vi "Iterate Owned Items.vi"(8 "Error In":errorcluster, 10 "Owned Items[]":refnum<vi>[](array[refnum]), 11 "Project Items In":T1[](array[typedef])) -> (0 "Error Out":errorcluster, 3 "Project Items Out":T1[](array[typedef]))   [LabVIEW 2014, in "i3-docs.lvlib"]
uses:
  i3-docs.lvlib
  Controls/project_item.ctl
  Controls/image_information.ctl
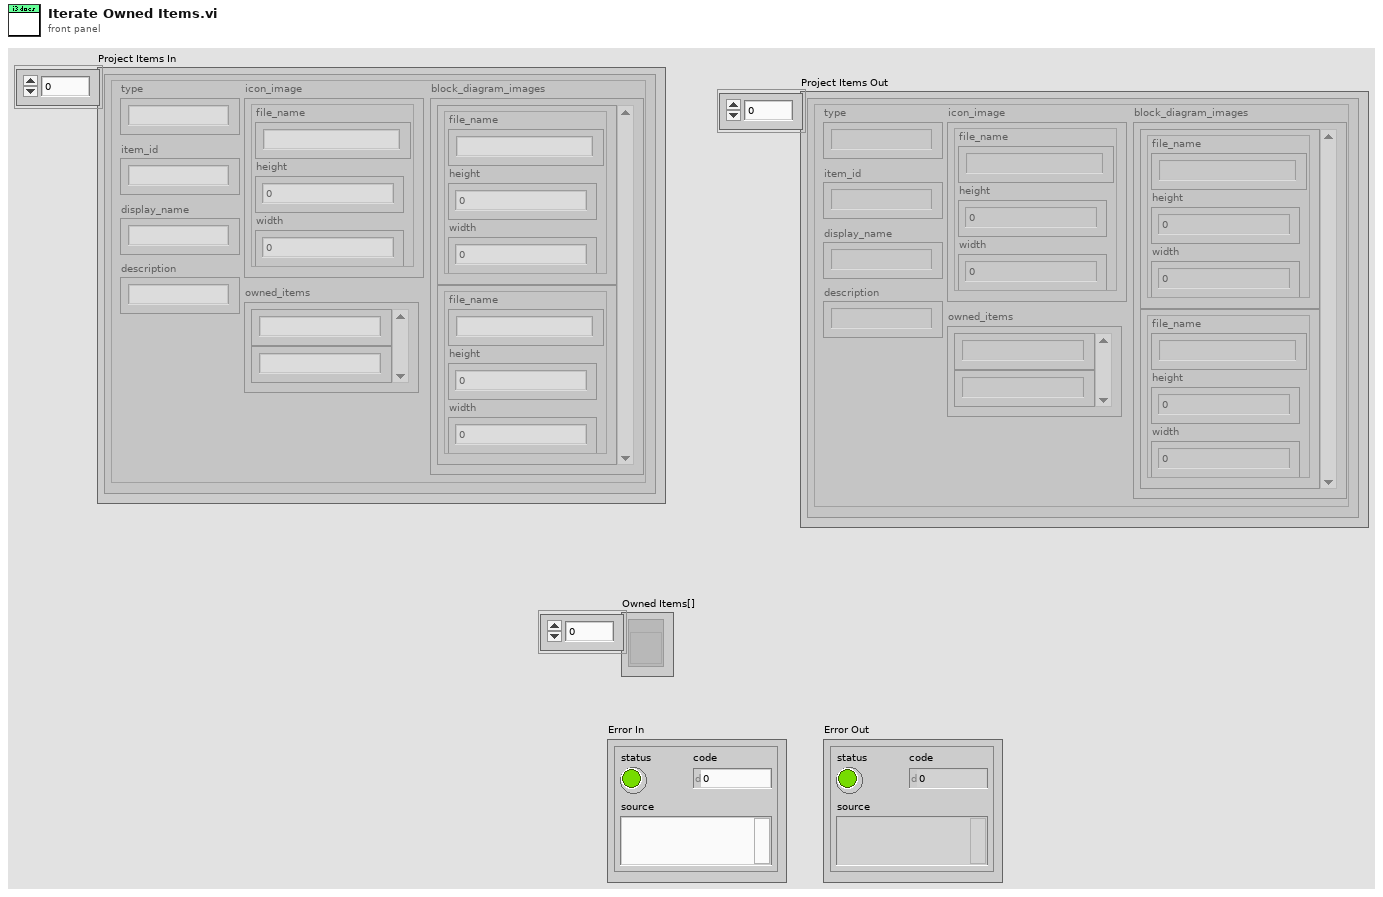
[diagram p1: front panel]
types:
  T1 = typedef "i3-docs.lvlib/project_item.ctl" = cluster{"type":string, "owned_items":string[], "item_id":string, "display_name":string, "description":string, "block_diagram_images":T2[], "icon_image":T2}
  T2 = typedef "i3-docs.lvlib/image_information.ctl" = cluster{"file_name":string, "height":i32, "width":i32}
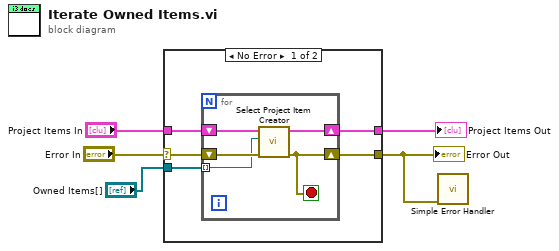
[diagram p0: block diagram]
diagram:
  n1 = case shown="No Error" "Error In" {
    selector: "Error In" -> [w10 w16]
    tunnel: "Project Items In" -> [w9 w17]
    tunnel: [w8 w16] -> w1
    tunnel: [w7 w17] -> w3
    tunnel: "Owned Items[]" -> [w6 _]
    frame No Error {
      n2 = for {
        tunnel: w6 -> [w11] mode=indexing
        shift-right: [w13] -> w8
        shift-left: w10 -> [w12]
        shift-right: [w14] -> w7
        shift-left: w9 -> [w15]
        stop <- w13 stop-if-true
        n3 = call "Select Project Item Creator.vi"("Error In"=w12, "ProjectItem Refnum"=w11, "Project Items In"=w15) -> ("Error Out"=w13:errorcluster, "Project Items Out"=w14:T1[])  [unwired: 7 in]
      }
    }
    frame Error {
    }
  }
  "Error Out" <- w1
  "Project Items Out" <- w3
  n4 = call <vilib>:"Simple Error Handler.vi"("error in (no error)"=w1) -> ()  [unwired: 4 in, 5 out]
